vi "goToNextTriple.vi"(4 "Samples":dbl, 6 "RobotModelAllInformation in":T1, 9 "triples (V0, Vf, V_sent)":dbl[][](array[numeric]), 10 "crash?":bool, 11 "Robot in":refnum<class "Robot.lvclass">) -> (3 "RobotModelAllInformation out":T1)   [LabVIEW 2020, in "Game.lvclass"]
uses:
  Game.lvclass
  Controls/RobotModelAllInformation.ctl
  Controls/RobotModel.ctl
  Controls/RobotModelTestCrashCase.ctl
  Robot_class/Robot.lvclass
  Robot_class/Robot.lvclass/Robot.ctl
  Robot_class/Read est_v_tang.vi
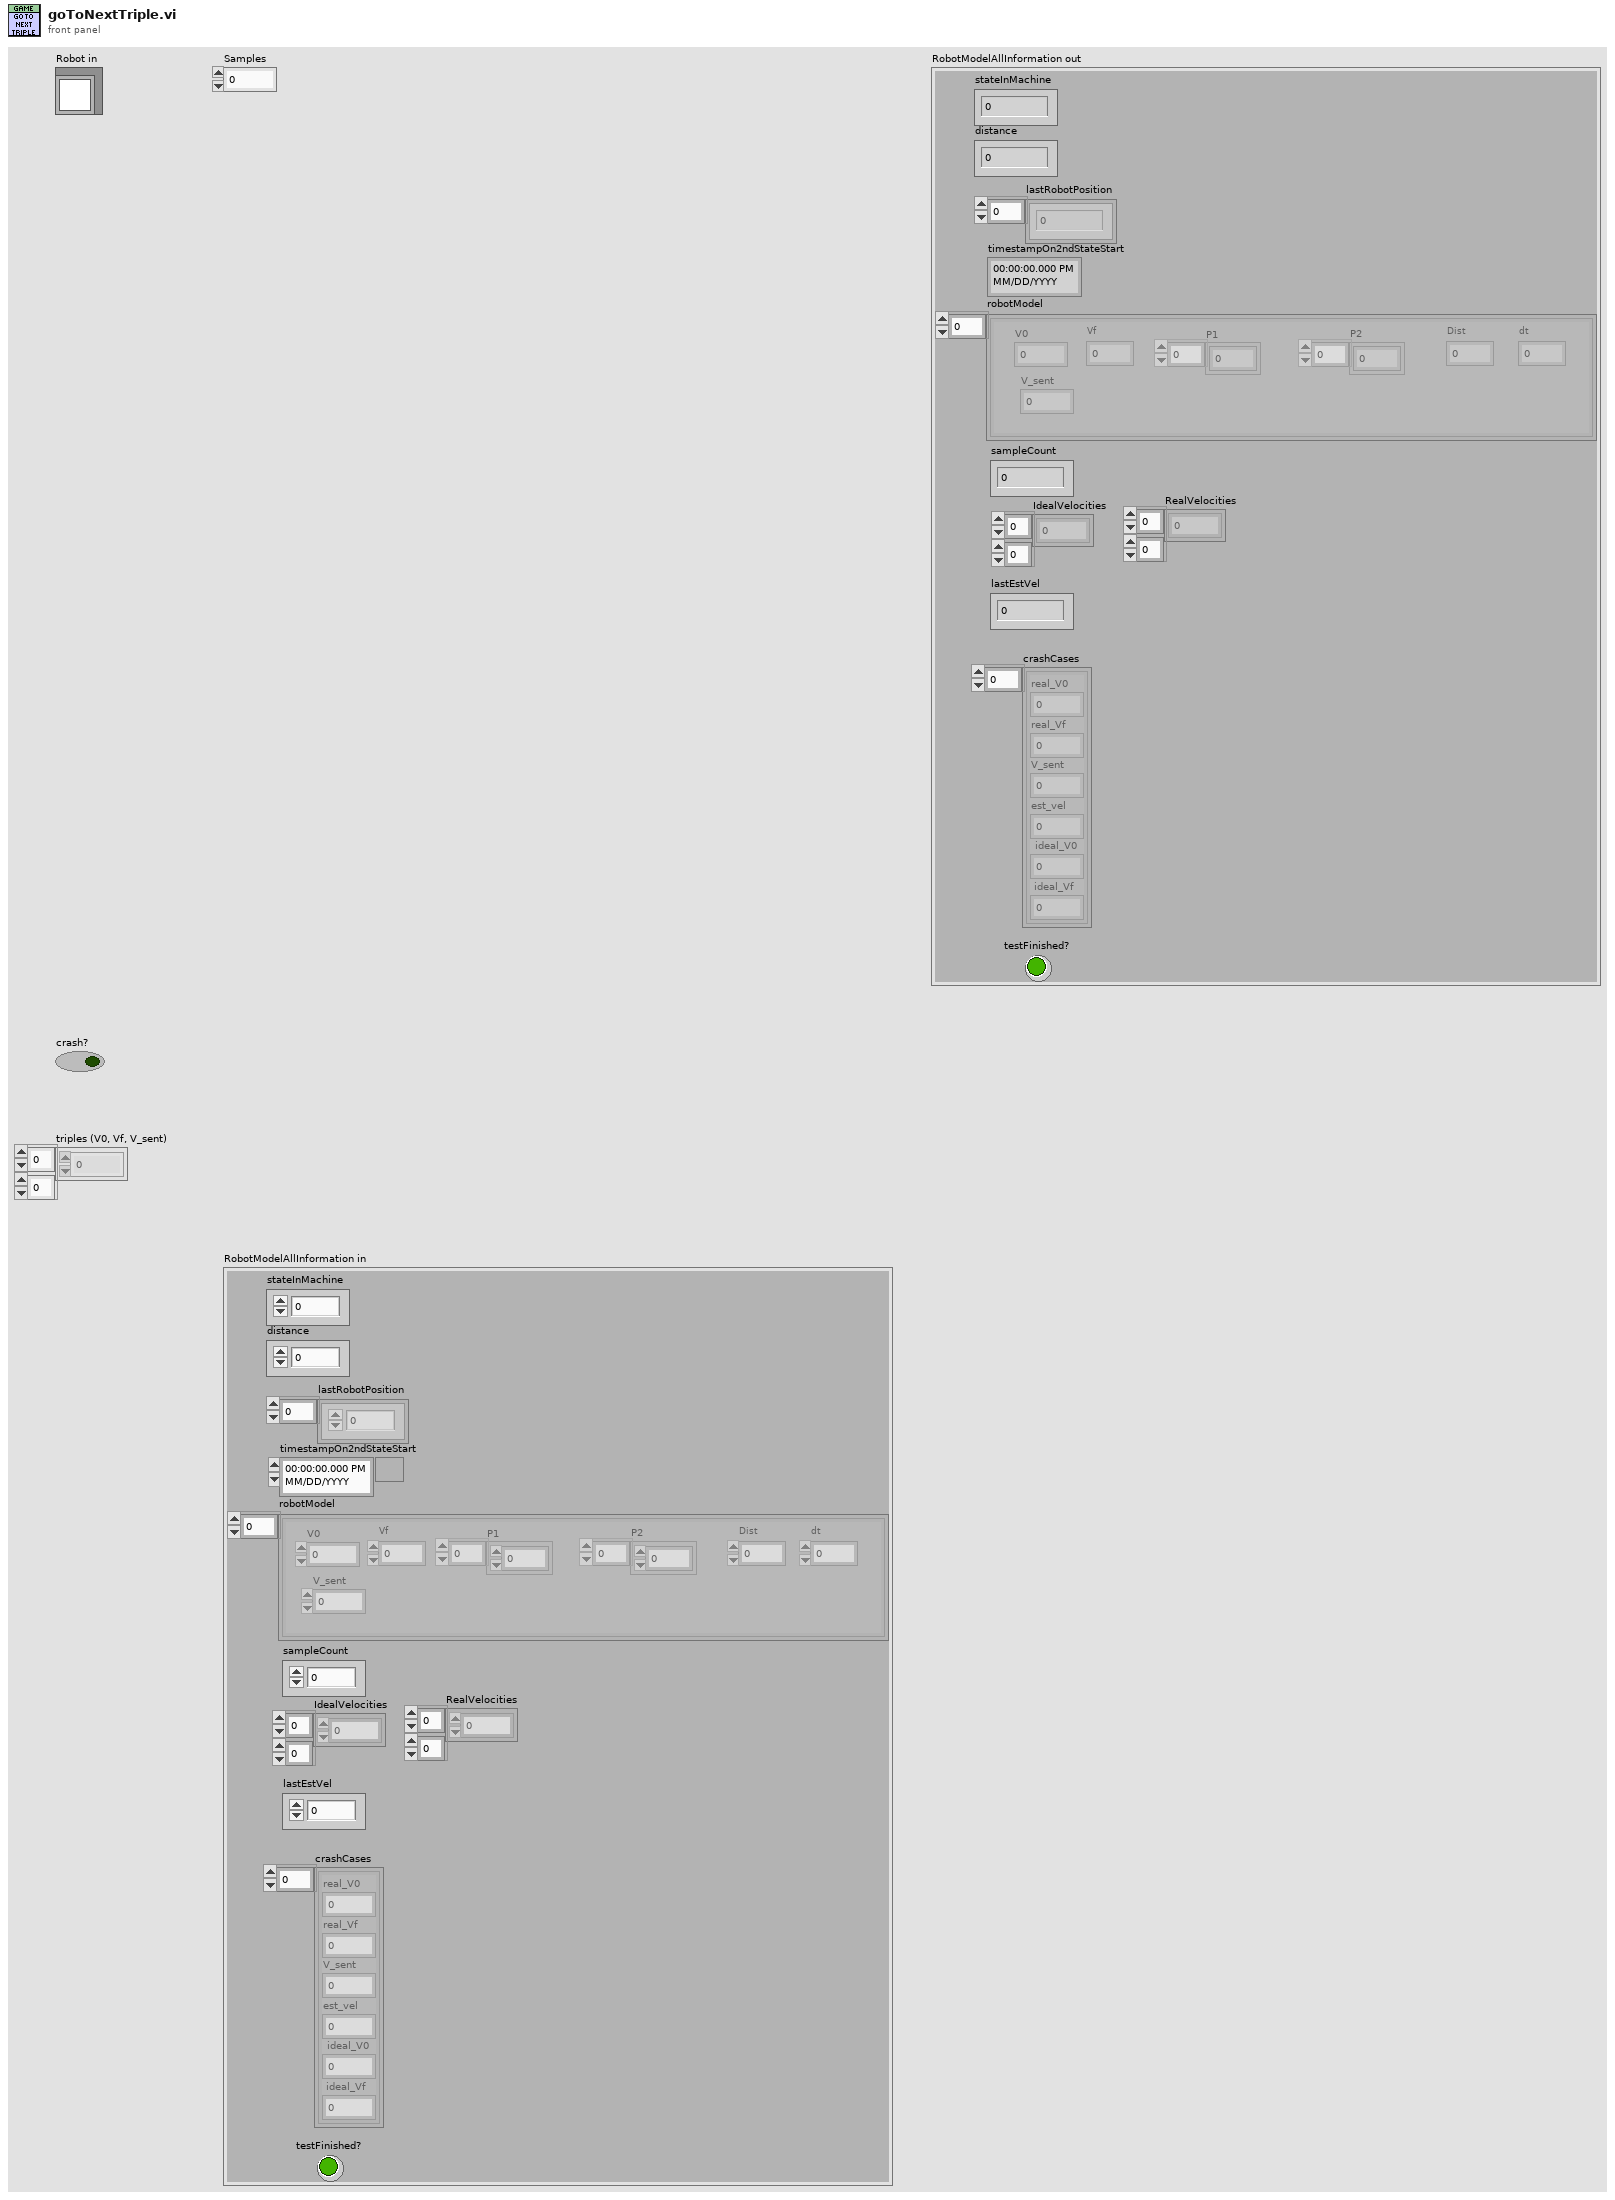
[diagram p1: front panel]
types:
  T1 = typedef "RobotModelAllInformation.ctl" = cluster{"distance":dbl, "lastRobotPosition":dbl[], "timestampOn2ndStateStart":timestamp, "robotModel":T2[], "sampleCount":i32, "stateInMachine":i32, "crashCases":T3[], "lastEstVel":dbl, "IdealVelocities":dbl[][], "RealVelocities":dbl[][], "testFinished?":bool}
  T2 = typedef "RobotModel.ctl" = cluster{"V0":dbl, "Vf":dbl, "Dist":dbl, "dt":dbl, "P1":dbl[], "P2":dbl[], "V_sent":dbl}
  T3 = typedef "RobotModelTestCrashCase.ctl" = cluster{"real_V0":dbl, "real_Vf":dbl, "V_sent":dbl, "est_vel":dbl, "ideal_V0":dbl, "ideal_Vf":dbl}
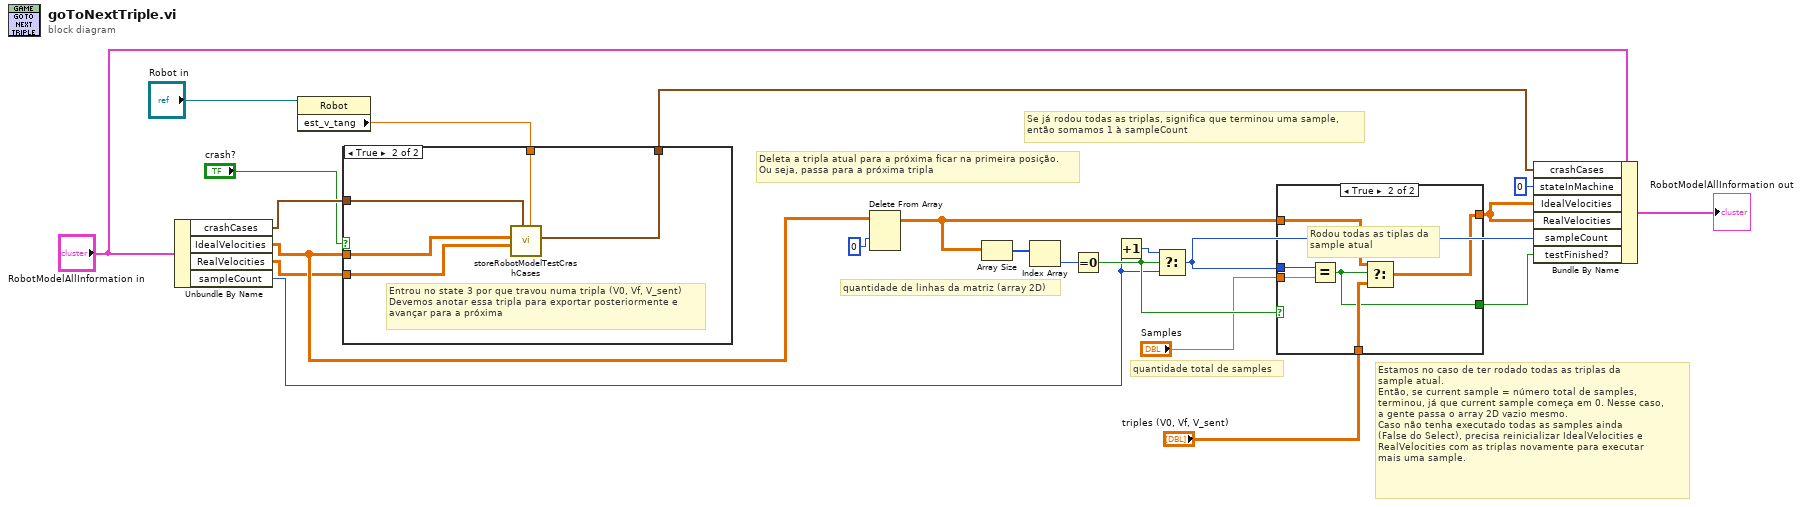
[diagram p0: block diagram]
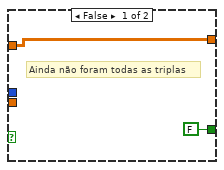
[diagram p3: hidden frame]
diagram:
  # "quantidade total de samples"
  # "Estamos no caso de ter rodado todas as triplas da\nsample atual.\nEntão, se current sample = número total de samples, \nterminou, já que current sample começa em 0. Nesse caso,\na gente passa o array 2D vazio mesmo.\nCaso não tenha executado todas as samples ainda\n(False do Select), precisa reinicializar IdealVelocities e\nRealVelocities com as triplas novamente para executar\nmais uma sample."
  # "Se já rodou todas as triplas, significa que terminou uma sample,\nentão somamos 1 à sampleCount"
  # "quantidade de linhas da matriz (array 2D)"
  # "Deleta a tripla atual para a próxima ficar na primeira posição.\nOu seja, passa para a próxima tripla"
  n1 = Unbundle By Name("RobotModelAllInformation in") -> ("crashCases"=w8:T3[], "IdealVelocities"=w10:dbl[][], "RealVelocities"=w9:dbl[][], "sampleCount"=w15:i32)
  n2 = property class="Robot"(reference="Robot in") -> ("est_v_tang"=w3:dbl)  [unwired: 1 in, 2 out]
  n3 = case shown="True" "crash?" {
    tunnel: w3 -> [_ w28]
    tunnel: [w23 w27] -> w6
    tunnel: w8 -> [w23 w24]
    tunnel: w10 -> [_ w26]
    tunnel: w9 -> [_ w25]
    frame False {
      # "Entrou em 3, mas não foi por causa de crash"
    }
    frame True {
      # "Entrou no state 3 por que travou numa tripla (V0, Vf, V_sent)\nDevemos anotar essa tripla para exportar posteriormente e\navançar para a próxima"
      n4 = call "storeRobotModelTestCrashCases.vi"("est_vel"=w28, "CrashCases"=w24, "RealVelocities"=w25, "IdealVelocities"=w26) -> ("CrashCasesArray out"=w27:T3[])  [unwired: 5 in, 2 out]
    }
  }
  n5 = Delete From Array(array=w10, index (row)=0) -> (array with subset deleted=w19:dbl[][])  [unwired: 2 in, 1 out]
  n6 = Array Size(array=w19) -> (size(s)=w12:i32[])
  n7 = Index Array(array=w12) -> (element=w13:i32)  [unwired: 1 in]
  n8 = Equal To 0?(x=w13) -> (x = 0?=w21:bool)
  n9 = Increment(x=w15) -> (x+1=w14:i32)
  n10 = Select(t=w14, s=w21, f=w15) -> (s? t:f=w16:i32)
  n11 = case shown="True" w21 {
    tunnel: w16 -> [_ w36]
    tunnel: "Samples" -> [_ w35]
    tunnel: "triples (V0, Vf, V_sent)" -> [_ w34]
    tunnel: w19 -> [w30 w33]
    tunnel: [w30 w32] -> w20
    tunnel: [FALSE w31] -> w22
    frame False {
      # "Ainda não foram todas as triplas"
    }
    frame True {
      # "Rodou todas as tiplas da\nsample atual"
      n12 = Equal?(x=w36, y=w35) -> (x = y?=w31:bool)
      n13 = Select(t=w33, s=w31, f=w34) -> (s? t:f=w32:dbl[][])
    }
  }
  n14 = Bundle By Name(cluster="RobotModelAllInformation in", "crashCases"=w6, "stateInMachine"=0, "IdealVelocities"=w20, "RealVelocities"=w20, "sampleCount"=w16, "testFinished?"=w22) -> (→"RobotModelAllInformation out":T1)
